vi "GlobalValves.vi"() -> ()   [LabVIEW 2012]
panel:
  in  "valves status":bool[](array[boolean])=[FALSE, FALSE, FALSE, FALSE, FALSE, FALSE, FALSE, FALSE]
  in  "valve open time":u32=1000
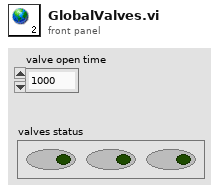
[diagram p1: front panel]
diagram:
